vi "Write Core.vi"(8 "error in (no error)":errorcluster, 10 "PV":refnum<class "PV.lvclass">, 11 "PVConnection in":refnum<class "SVConnection.lvclass">) -> (0 "error out":errorcluster, 3 "PVConnection out":refnum<class "SVConnection.lvclass">)   [LabVIEW 2015, in "CS++ProcessVariables.lvlib" / "SVConnection.lvclass"]
doc: "Publish a process variable."
uses:
  SVConnection.lvclass
  ProcessVariable/PV.lvclass
  ProcessVariable/PV.lvclass/PV.ctl
  SVConnection.lvclass/SVConnection.ctl
  Libraries/Utilities/CS++Utilities.lvlib
  PVConnection/PVConnection.lvclass
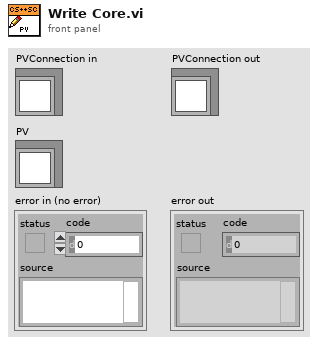
[diagram p1: front panel]
types:
  T1 = cluster{"Read Access":enum8{"Allowed", "Required", "None"}, "Write Access":enum8{"Allowed", "Required", "None"}}
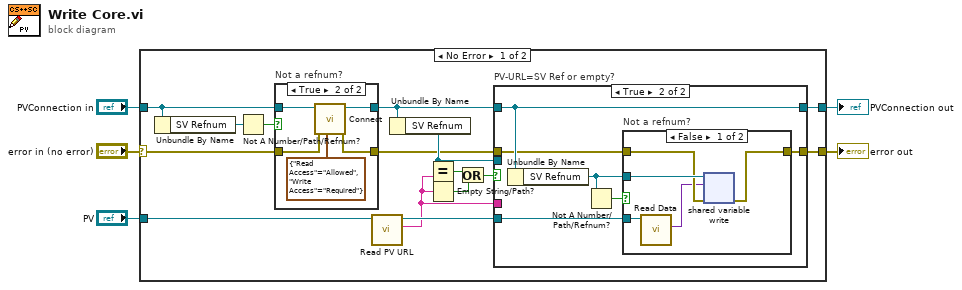
[diagram p0: block diagram]
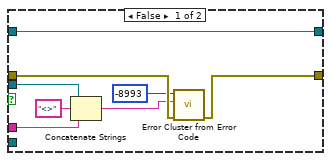
[diagram p3: hidden frame]
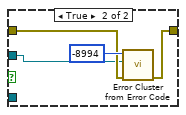
[diagram p4: hidden frame]
diagram:
  n1 = case shown="No Error" "error in (no error)" {
    selector: "error in (no error)" -> [w8 w52]
    tunnel: [w20 w52] -> w5
    tunnel: [w19 w51] -> w4
    tunnel: "PV" -> [w18 _]
    tunnel: "PVConnection in" -> [w7 w51]
    frame No Error {
      n2 = Unbundle By Name(w7) -> ("SV Refnum"=w10:refnum<k21>)
      n3 = Not A Number/Path/Refnum?(number/path/refnum=w10) -> (NaN/Path/Refnum?=w11:bool)
      n4 = case "Not a refnum?" shown="True" w11 {
        tunnel: w7 -> [w21 w27]
        tunnel: [w21 w26] -> w6
        tunnel: w8 -> [w22 w25]
        tunnel: [w22 w24] -> w9
        frame False {
        }
        frame True {
          n5 = call "Connect.vi"("Access (R/W allowed)"=T1 {"Read Access"=enum."Allowed", "Write Access"=enum."Required"}, "Error In"=w25, "PVConnection in"=w27) -> ("Error Out"=w24:errorcluster, "PVConnection out"=w26:refnum<class "SVConnection.lvclass">)  [unwired: 7 in]
        }
      }
      n6 = call "Read PV URL.vi"("PV in"=w18) -> ("PV URL"=w12:string, "PV out"=w15:refnum<class "PV.lvclass">)  [unwired: 8 in, 1 out]
      n7 = Unbundle By Name(w6) -> ("SV Refnum"=w13:refnum<k21>)
      n8 = Equal?(x=w13, y=w12) -> (x = y?=w16:bool)
      n9 = Empty String/Path?(string/path=w12) -> (empty?=w17:bool)
      n10 = Or(x=w16, y=w17) -> (x .or. y?=w14:bool)
      n11 = case "PV-URL=SV Ref or empty?" shown="True" w14 {
        tunnel: [w33 w39] -> w20
        tunnel: [w35 w41] -> w19
        tunnel: w6 -> [w35 w41]
        tunnel: w9 -> [w34 w40]
        tunnel: w15 -> [_ w38]
        tunnel: w13 -> [w31 _]
        tunnel: w12 -> [w30 _]
        frame False {
          n12 = Concatenate Strings(w31, "<>" ("string"), w30) -> (w28:string)
          n13 = call "Error Cluster from Error Code.vi"("Error In"=w34, "Error Message (\"\")"=w28, "Error Code (0)"=-8993 ("error code (0)")) -> ("Error Out"=w33:errorcluster)  [unwired: 8 in]
        }
        frame True {
          n14 = Unbundle By Name(w41) -> ("SV Refnum"=w36:refnum<k21>)
          n15 = Not A Number/Path/Refnum?(number/path/refnum=w36) -> (NaN/Path/Refnum?=w37:bool)
          n16 = case "Not a refnum?" shown="False" w37 {
            tunnel: w36 -> [w46 w47]
            tunnel: w40 -> [w45 w49]
            tunnel: [w44 w48] -> w39
            tunnel: w38 -> [w42 _]
            frame False {
              n17 = call "Read Data.vi"("PV in"=w42) -> ("Data"=w43:variant)  [unwired: 8 in, 2 out]
              n18 = shared-variable-write(w46, w45, w43) -> (w44:errorcluster)  [unwired: 1 out]
            }
            frame True {
              n19 = call "Error Cluster from Error Code.vi"("Error In"=w49, "Error Message (\"\")"=w47, "Error Code (0)"=-8994 ("error code (0)")) -> ("Error Out"=w48:errorcluster)  [unwired: 8 in]
            }
          }
        }
      }
    }
    frame Error {
    }
  }
  "error out" <- w5
  "PVConnection out" <- w4
